vi "Simple UDP - Sender_and_receiver.vi"() -> ()   [LabVIEW 2013]
doc: "The UDP protocol differs from TCP in that there is no error-checking with the packets of information that are sent, and thus no guarantee whatsoever that an intended recipient will actually receive a given piece of data.\n\nUDP does offer the ability to \"broadcast\" data across a network--simply specify an IP Address of all ones (255.255.255.255) to attempt to broadcast information network-wide. Keep in mind that routers and other network hardware will generally refuse to forward the broadcast beyond certain points, so the extent of the broadcast will in practice be limited."
panel:
  out "Received data":string[](array[string])
  out "Data Sent":string
  in  "Stop":bool
  # "Overview: Demonstrates the use of the UDP functions to send data over a UDP connection.\nInstructions:\n1. Run the VI.\n2. Open Simple UDP - Receiver.vi and follow the instructions on its front panel.\n3. Click Stop to stop the VI."
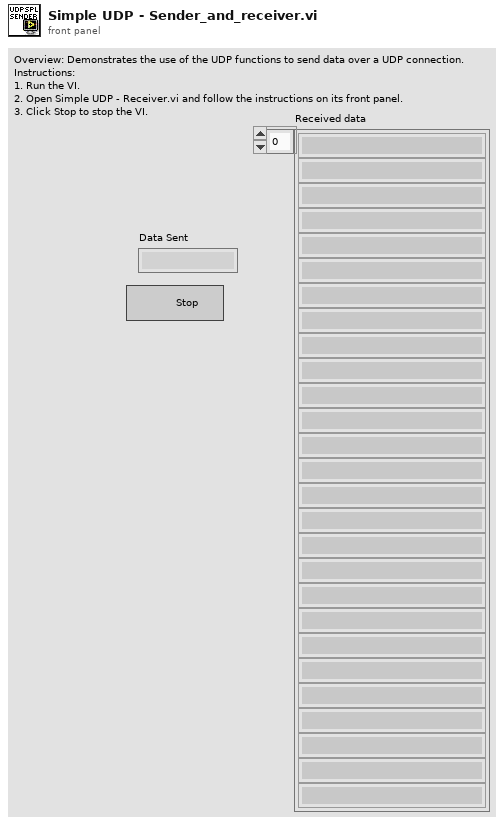
[diagram p1: front panel]
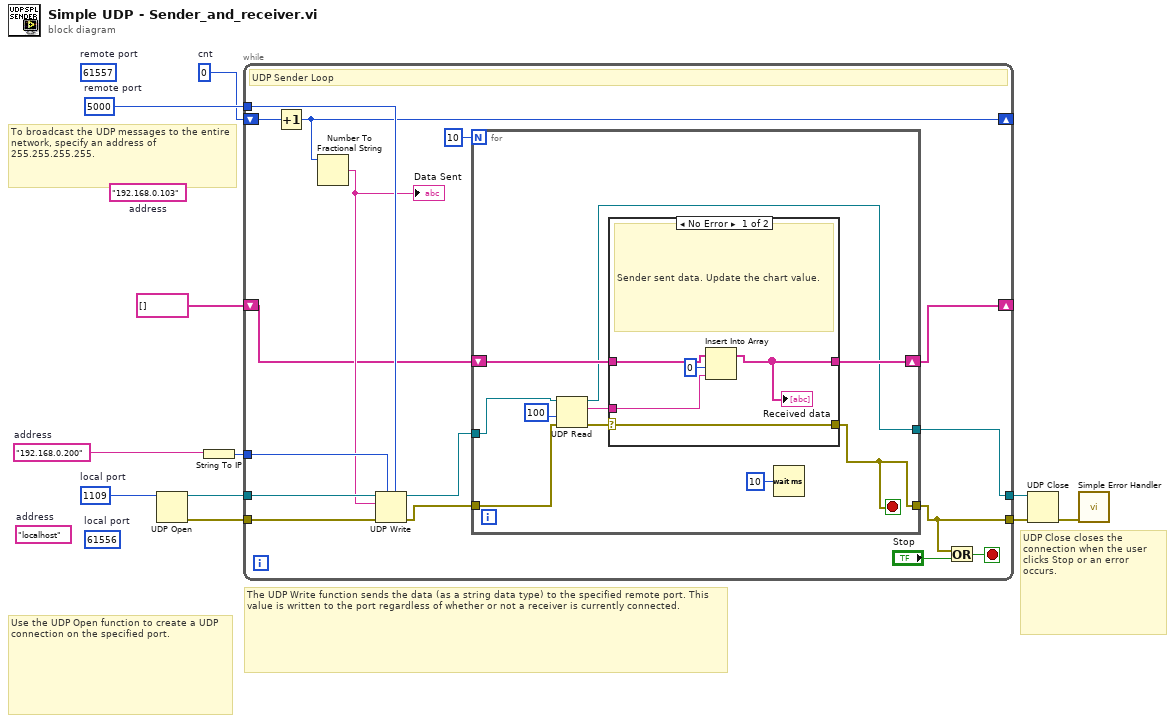
[diagram p0: block diagram]
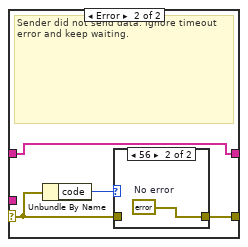
[diagram p2: hidden frame]
diagram:
  (unwired) "192.168.0.103"  # address
  w3 = u16 0  # cnt
  (unwired) u16 61557  # remote port
  (unwired) u16 61556  # local port
  w2 = "192.168.0.200"  # address
  w4 = u16 5000  # remote port
  w5 = u16 1109  # local port
  (unwired) "localhost"  # address
  # "To broadcast the UDP messages to the entire network, specify an address of 255.255.255.255."
  # "UDP Close closes the connection when the user clicks Stop or an error occurs."
  # "The UDP Write function sends the data (as a string data type) to the specified remote port. This value is written to the port regardless of whether or not a receiver is currently connected."
  # "Use the UDP Open function to create a UDP connection on the specified port."
  n1 = UDP Open(11:w5) -> (port=w7:refnum<k16>, 0:w6:errorcluster)  [unwired: 4 in, 1 out]
  n2 = String To IP(1:w2) -> (0:w8:u32)
  n3 = while {
    tunnel: [w17] -> w10
    tunnel: w7 -> [w27]
    tunnel: w6 -> [w26]
    tunnel: [w13] -> w11
    tunnel: w8 -> [w23]
    tunnel: w4 -> [w22]
    shift-right: [w20] -> _
    shift-left: w3 -> [w21]
    shift-right: [w12] -> _
    shift-left: string[] [] ("Array 2") -> [w15]
    stop <- w25 stop-if-true
    # "UDP Sender Loop"
    n4 = Increment(x=w21) -> (x+1=w20:u16)
    n5 = Number To Fractional String(number=w20) -> (F-format string=w19:string)  [unwired: 3 in]
    "Data Sent" <- w19
    n6 = UDP Write(address=w23, port or service name=w22, connection ID=w27, data in=w19, 8:w26) -> (error out=w18:errorcluster, 3:w16:refnum<k16>)  [unwired: 1 in]
    n7 = for {
      N: 10 -> [_]
      tunnel: w18 -> [w30]
      tunnel: [w28] -> w17
      tunnel: w16 -> [w31]
      shift-right: [w32] -> w12
      shift-left: w15 -> [w33]
      tunnel: [w29] -> w13
      stop <- w28 stop-if-true
      n8 = UDP Read(connection ID=w31, timeout ms (25000)=100, 8:w30) -> (data out=w35:string, error out=w34:errorcluster, 3:w29:refnum<k16>)  [unwired: 3 out]
      n9 = case shown="No Error" w34 {
        selector: w34 -> [w42 w45]
        tunnel: w35 -> [w39 _]
        tunnel: [w42 w44] -> w28
        tunnel: w33 -> [w41 w43]
        tunnel: [w38 w43] -> w32
        frame No Error {
          # "Sender sent data. Update the chart value."
          n10 = Insert Into Array(array=w41, index=0, new element=w39) -> (w38:string[])
          "Received data" <- w38
        }
        frame Error {
          # "Sender did not send data. Ignore timeout error and keep waiting."
          n11 = Unbundle By Name(w45) -> ("code"=w46:i32)
          n12 = case shown="56" w46 {
            tunnel: w45 -> [w47 _]
            tunnel: [w47 w48] -> w44
            frame Default {
            }
            frame 56 {
              w48 = errorcluster {"status"=FALSE, "code"=0, "source"=""}  # No error
            }
          }
        }
      }
      n13 = Wait (ms)(milliseconds to wait=u32 10) -> ()  [unwired: 1 out]
    }
    n14 = Or(x=w17, y="Stop") -> (x .or. y?=w25:bool)
  }
  n15 = UDP Close(connection ID=w11, 8:w10) -> (error out=w9:errorcluster)  [unwired: 1 out]
  n16 = call <vilib>:"Simple Error Handler.vi"("error in (no error)"=w9) -> ()  [unwired: 4 in, 5 out]
